vi "CSDB_Config.get ClassNames.vi"(5 "error in (no error)":errorcluster) -> (17 "ClassNames":string[](array[string]), 19 "error out":errorcluster)   [LabVIEW 2014, in "CSDB_Config.lvlib"]
doc: "Gets the name of all classes registered in the database."
uses:
  CSDB_Config.lvlib
  <vilib>/addons/database/_DB Variant To Data/Database Variant To Data.xnode
  <vilib>/addons/database/NI_Database_API.lvlib
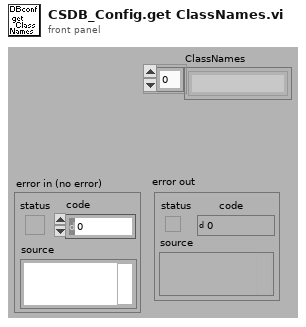
[diagram p1: front panel]
types:
  T1 = typedef "NI_Database_API.lvlib/Conn ObjectReference.ctl" = refnum<k1>
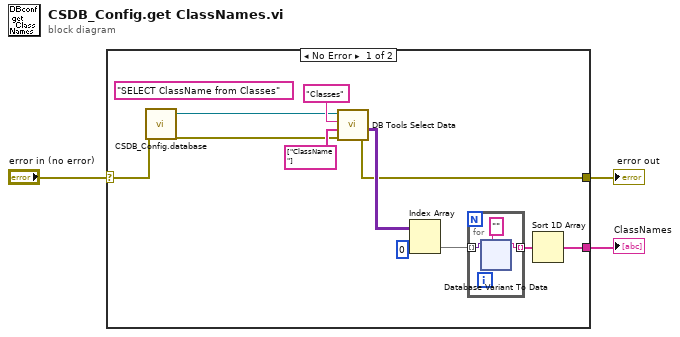
[diagram p0: block diagram]
diagram:
  n1 = case shown="No Error" "error in (no error)" {
    selector: "error in (no error)" -> [w6 w50]
    tunnel: [w13 _] -> w3
    tunnel: [w7 w50] -> w2
    frame No Error {
      (unwired) "SELECT ClassName from Classes" ("SQL statement")
      n2 = call "CSDB_Config.database.vi"("error in (no error)"=w6) -> ("connectionRef out"=w4:T1, "error out"=w5:errorcluster)  [unwired: 17 in]
      n3 = call <vilib>:"DB Tools Select Data.vi"("error in (no error)"=w5, "columns"=string[] ["ClassName"], "table"="Classes", "connection reference"=w4) -> ("error out"=w7:errorcluster, "data"=w10:variant[][])  [unwired: 2 in, 1 out]
      n4 = Index Array(array=w10, index (col)=0 ("disabled index (col)")) -> (element=w9:variant[])  [unwired: 1 in]
      n5 = for {
        tunnel: w9 -> [w17] mode=indexing
        tunnel: [w16] -> w8 mode=indexing
        n6 = xnode "Database Variant To Data"("database variant"=w17, "type"="") -> ("data"=w16:string)  [unwired: 1 in, 1 out]
      }
      n7 = Sort 1D Array(array=w8) -> (sorted array=w13:string[])
    }
    frame Error {
    }
  }
  "error out" <- w2
  "ClassNames" <- w3
